vi "PID test.vi"(6 "PID gains":T1={"proportional gain (Kc)"=60.0, "integral time (Ti, min)"=0.2, "derivative time (Td, min)"=0.0}, 10 "PV deg C":dbl format="%.2f", 11 "User SP Deg C":dbl format="%.2f") -> (2 "output V":dbl format="%.2f")   [LabVIEW 2011]
uses:
  <vilib>/addons/control/pid/pid.llb/PID (DBL).vi
  <vilib>/addons/control/pid/NI_PID_pid.lvlib
panel:
  out "output":dbl format="%.2f"
  in  "stop":bool
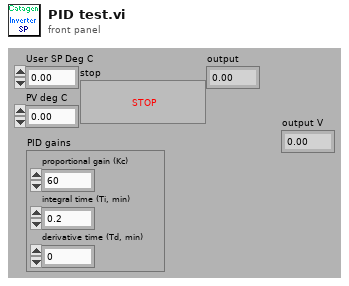
[diagram p1: front panel]
types:
  T1 = cluster{"proportional gain (Kc)":dbl, "integral time (Ti, min)":dbl, "derivative time (Td, min)":dbl}
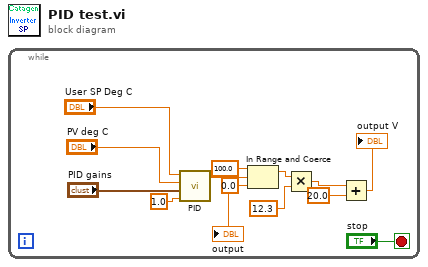
[diagram p0: block diagram]
diagram:
  n1 = while {
    stop <- "stop" stop-if-true
    n2 = call-poly <vilib>:"PID.vi"("dt (s)"=1.0, "PID gains"="PID gains", "process variable"="PV deg C", "setpoint"="User SP Deg C") -> ("output"=w10:dbl)  [unwired: 6 in, 1 out]
    "output" <- w10
    n3 = In Range and Coerce(upper limit=100.0, x=w10, lower limit=0.0) -> (coerced(x)=w6:dbl)  [unwired: 1 out]
    n4 = Multiply(x=w6, y=12.3) -> (x*y=w4:dbl)
    n5 = Add(x=w4, y=20.0) -> (x+y=→"output V":dbl)
  }
